vi "Tx to UDP.vi"(6 "Header Details.CustomHeaderLogic":T1, 7 "Data Conversion":T2, 8 "error in (no error)":errorcluster, 10 "Tx Array":dbl[](array[numeric]), 11 "Header Info":bool[](array[boolean])) -> (0 "error out":errorcluster, 1 "payload":dbl[](array[numeric]), 2 "Tx String":string, 5 "Data Conversion out":T2)   [LabVIEW 2019, in "UDP-Custom-Device Engine.lvlib"]
uses:
  UDP-Custom-Device Engine.lvlib
  Types/Engine - Data Conversion Config.ctl
  <vilib>/NI VeriStand/VeriStand Data/Byte Buffer/Byte Buffer.lvclass
  <vilib>/NI VeriStand/VeriStand Data/Byte Buffer/Byte Buffer.Mapping.ctl
  <vilib>/NI VeriStand/VeriStand Data/Typedefs/Typedefs.Data Types.ctl
  Shared/Types/Shared - Custom Header.ctl
  <vilib>/NI VeriStand/VeriStand Data/Byte Buffer/Byte Buffer.lvclass/Byte Buffer.ctl
  <vilib>/NI VeriStand/VeriStand Data/Pointer Operations/Pointer.Write (DBL).vi
  <vilib>/NI VeriStand/VeriStand Data/Byte Buffer/Byte Buffer.Read (String).vi
  <vilib>/NI VeriStand/VeriStand Data/Memory Management/Memory Management.MoveDblBlock.Write (Double).vi
  <vilib>/NI VeriStand/VeriStand Data/Byte Buffer/Byte Buffer.Write.Typed Double Array.vi
  <vilib>/NI VeriStand/VeriStand Data/Utilities/Utilities.Buffer.Double.vi
  <vilib>/NI VeriStand/VeriStand Data/Byte Buffer/Byte Buffer.Subset.Get.vi
  <vilib>/NI VeriStand/VeriStand Data/Byte Buffer/Byte Buffer.Write.vi
  <vilib>/NI VeriStand/VeriStand Data/Byte Buffer/Byte Buffer.Write (1D Boolean).vi
  <vilib>/NI VeriStand/VeriStand Data/Type Conversion/Type Conversion.From Double.Subset.vi
  <vilib>/NI VeriStand/VeriStand Data/Type Conversion/Type Conversion.From Double.Subset (1D Boolean).vi
  <vilib>/NI VeriStand/VeriStand Data/Byte Buffer/Byte Buffer.Write (1D SGL).vi
  <vilib>/NI VeriStand/VeriStand Data/Type Conversion/Type Conversion.From Double.Subset (1D SGL).vi
  <vilib>/NI VeriStand/VeriStand Data/Byte Buffer/Byte Buffer.Write (1D DBL).vi
  <vilib>/NI VeriStand/VeriStand Data/Byte Buffer/Byte Buffer.Write (1D I8).vi
  <vilib>/NI VeriStand/VeriStand Data/Type Conversion/Type Conversion.From Double.Subset (1D I8).vi
  <vilib>/NI VeriStand/VeriStand Data/Byte Buffer/Byte Buffer.Write (1D I16).vi
  <vilib>/NI VeriStand/VeriStand Data/Type Conversion/Type Conversion.From Double.Subset (1D I16).vi
  <vilib>/NI VeriStand/VeriStand Data/Byte Buffer/Byte Buffer.Write (1D I32).vi
  <vilib>/NI VeriStand/VeriStand Data/Type Conversion/Type Conversion.From Double.Subset (1D I32).vi
  <vilib>/NI VeriStand/VeriStand Data/Byte Buffer/Byte Buffer.Write (1D I64).vi
  <vilib>/NI VeriStand/VeriStand Data/Type Conversion/Type Conversion.From Double.Subset (1D I64).vi
  <vilib>/NI VeriStand/VeriStand Data/Byte Buffer/Byte Buffer.Write (1D U8).vi
  <vilib>/NI VeriStand/VeriStand Data/Type Conversion/Type Conversion.From Double.Subset (1D U8).vi
  <vilib>/NI VeriStand/VeriStand Data/Byte Buffer/Byte Buffer.Write (1D U16).vi
  <vilib>/NI VeriStand/VeriStand Data/Type Conversion/Type Conversion.From Double.Subset (1D U16).vi
  <vilib>/NI VeriStand/VeriStand Data/Byte Buffer/Byte Buffer.Write (1D U32).vi
  <vilib>/NI VeriStand/VeriStand Data/Type Conversion/Type Conversion.From Double.Subset (1D U32).vi
  <vilib>/NI VeriStand/VeriStand Data/Byte Buffer/Byte Buffer.Write (1D U64).vi
  <vilib>/NI VeriStand/VeriStand Data/Type Conversion/Type Conversion.From Double.Subset (1D U64).vi
  <vilib>/NI VeriStand/VeriStand Data/Memory Management/Memory Management.MoveByteBlock.Write (String).vi
  <vilib>/NI VeriStand/VeriStand Data/Byte Buffer/Byte Buffer.Get Buffer Pointer.vi
  <vilib>/NI VeriStand/VeriStand Data/Byte Buffer/Byte Buffer.Write (String).vi
  <vilib>/NI VeriStand/VeriStand Data/Type Conversion/Type Conversion.From Double.vi
  <vilib>/NI VeriStand/VeriStand Data/Type Conversion/Type Conversion.From Double (1D Boolean).vi
  <vilib>/NI VeriStand/VeriStand Data/Type Conversion/Type Conversion.From Double (1D SGL).vi
  <vilib>/NI VeriStand/VeriStand Data/Type Conversion/Type Conversion.From Double (1D I8).vi
  <vilib>/NI VeriStand/VeriStand Data/Type Conversion/Type Conversion.From Double (1D I16).vi
  <vilib>/NI VeriStand/VeriStand Data/Type Conversion/Type Conversion.From Double (1D I32).vi
  <vilib>/NI VeriStand/VeriStand Data/Type Conversion/Type Conversion.From Double (1D I64).vi
  <vilib>/NI VeriStand/VeriStand Data/Type Conversion/Type Conversion.From Double (1D U8).vi
  <vilib>/NI VeriStand/VeriStand Data/Type Conversion/Type Conversion.From Double (1D U16).vi
  <vilib>/NI VeriStand/VeriStand Data/Type Conversion/Type Conversion.From Double (1D U32).vi
  <vilib>/NI VeriStand/VeriStand Data/Type Conversion/Type Conversion.From Double (1D U64).vi
  <vilib>/NI VeriStand/VeriStand Data/Byte Buffer/Byte Buffer.Subset.Set.vi
  <vilib>/NI VeriStand/VeriStand Data/Memory Management/Memory Management.MoveByteBlock.Read (String).vi
  <vilib>/NI VeriStand/VeriStand Data/Memory Management/Memory Management.Handle Return.vi
  <vilib>/NI VeriStand/VeriStand Data/Byte Buffer/Byte Buffer.Get Byte Order.vi
  <vilib>/NI VeriStand/VeriStand Data/VeriStand Data.lvlib
  Shared/UDP-Custom-Device Shared.lvlib
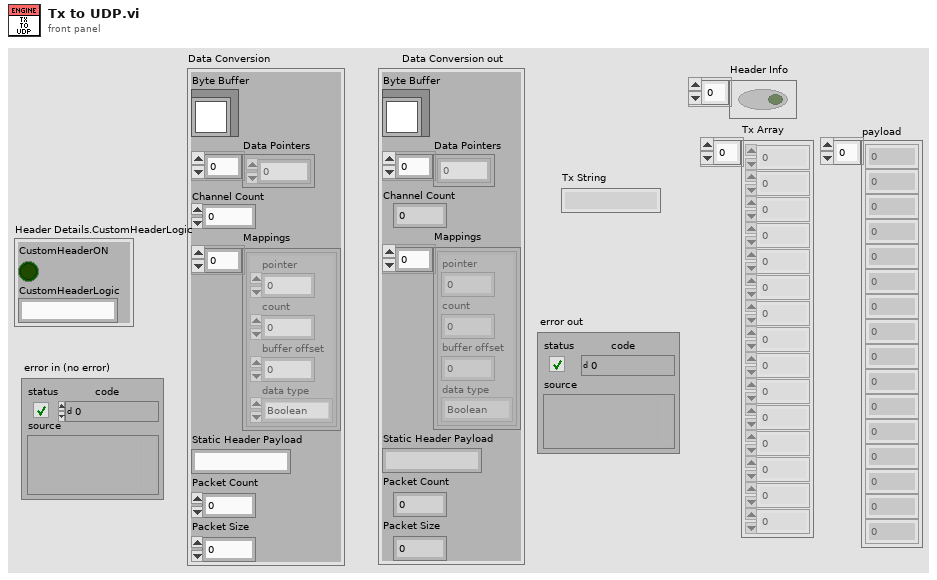
[diagram p1: front panel]
types:
  T1 = typedef "UDP-Custom-Device Shared.lvlib/Shared - Custom Header.ctl" = cluster{"CustomHeaderON":bool, "CustomHeaderLogic":string}
  T2 = typedef "UDP-Custom-Device Engine.lvlib/Engine - Data Conversion Config.ctl" = cluster{"Byte Buffer":refnum<class "Byte Buffer.lvclass">, "Data Pointers":u64[], "Channel Count":i32, "Mappings":T3[], "Static Header Payload":string, "Packet Count":dbl, "Packet Size":i32}
  T3 = typedef "VeriStand Data.lvlib/Byte Buffer.lvclass/Byte Buffer.Mapping.ctl" = cluster{"pointer":u64, "count":i64, "buffer offset":u64, "data type":T4}
  T4 = typedef "VeriStand Data.lvlib/Typedefs.Data Types.ctl" = enum16{"Boolean", "Single", "Double", "I8", "I16", "I32", "I64", "U8", "U16", "U32", "U64"}
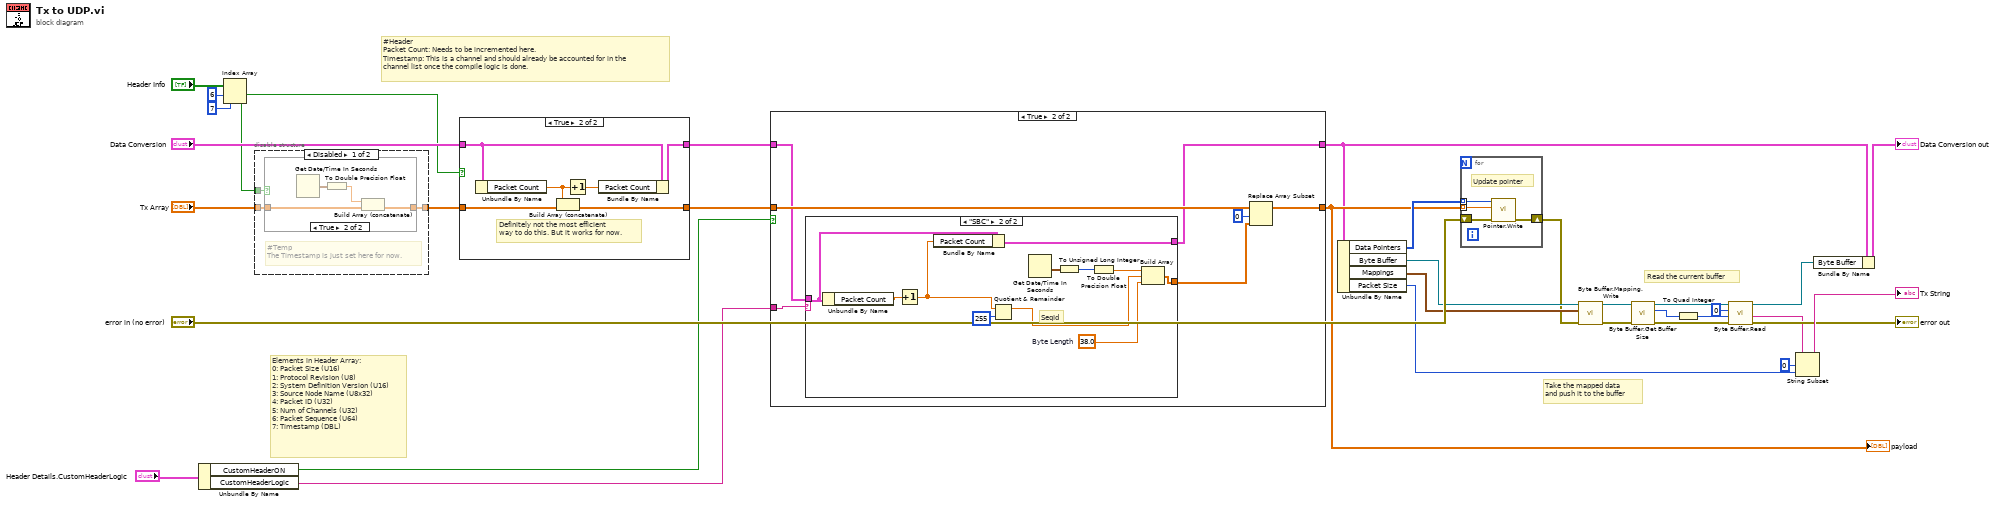
[diagram p0: block diagram]
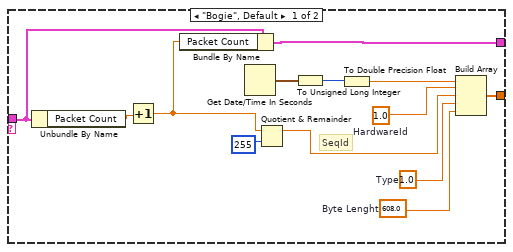
[diagram p3: hidden frame]
diagram:
  # "Elements in Header Array:\n0: Packet Size (U16)\n1: Protocol Revision (U8)\n2: System Definition Version (U16)\n3: Source Node Name (U8x32)\n4: Packet ID (U32)\n5: Num of Channels (U32)\n6: Packet Sequence (U64)\n7: Timestamp (DBL)"
  # "Read the current buffer"
  # "Take the mapped data\nand push it to the buffer"
  # "#Header\nPacket Count: Needs to be incremented here.\nTimestamp: This is a channel and should already be accounted for in the\nchannel list once the compile logic is done."
  n1 = Unbundle By Name("Header Details.CustomHeaderLogic") -> ("CustomHeaderON"=w6:bool, "CustomHeaderLogic"=w5:string)
  n2 = Index Array(array="Header Info", index #1=6 ("index"), index #2=7 ("index")) -> (element #1=w25:bool, element #2=w24:bool)
  n3 = disable-structure shown="Disabled" {
    disable-tunnel: w24 -> [w37 _]
    disable-tunnel: "Tx Array" -> [w36 w43]
    disable-tunnel: [w35 w43] -> w22
    frame Disabled {
      # "#Temp\nThe Timestamp is just set here for now."
      n4 = case shown="True" w37 {
        tunnel: [w38 w41] -> w35
        tunnel: w36 -> [w38 w42]
        frame False {
        }
        frame True {
          n5 = Get Date/Time In Seconds() -> (seconds since 1Jan1904=w40:timestamp)
          n6 = To Double Precision Float(number=w40) -> (double precision float=w39:dbl)
          n7 = Build Array (concatenate)(w39, w42) -> (w41:dbl[])
        }
      }
    }
    frame Enabled {
      # "Timestamp is an input channel\nat compile."
    }
  }
  n8 = case shown="True" w25 {
    tunnel: "Data Conversion" -> [w45 w51]
    tunnel: [w45 w50] -> w2
    tunnel: [w44 w46] -> w4
    tunnel: w22 -> [w44 w47]
    frame False {
    }
    frame True {
      # "Definitely not the most efficient\nway to do this. But it works for now."
      n9 = Unbundle By Name(w51) -> ("Packet Count"=w48:dbl)
      n10 = Build Array (concatenate)(w48, w47) -> (w46:dbl[])
      n11 = Increment(x=w48) -> (x+1=w49:dbl)
      n12 = Bundle By Name(cluster=w51, "Packet Count"=w49) -> (w50:T2)
    }
  }
  n13 = case shown="True" w6 {
    tunnel: w5 -> [_ w59]
    tunnel: w4 -> [w53 w57]
    tunnel: [w53 w60] -> w3
    tunnel: w2 -> [w52 w55]
    tunnel: [w52 w54] -> w1
    frame False {
    }
    frame True {
      n14 = case shown="\"SBC\"" w59 {
        tunnel: [w73 w84] -> w58
        tunnel: w55 -> [w69 w80]
        tunnel: [w68 w79] -> w54
        frame "Bogie", Default {
          w65 = 608.0  # Byte Lenght
          w66 = 1.0  # Type
          w67 = 1.0  # HardwareId
          # "SeqId"
          n15 = Unbundle By Name(w69) -> ("Packet Count"=w70:dbl)
          n16 = Increment(x=w70) -> (x+1=w64:dbl)
          n17 = Bundle By Name(cluster=w69, "Packet Count"=w64) -> (w68:T2)
          n18 = Get Date/Time In Seconds() -> (seconds since 1Jan1904=w63:timestamp)
          n19 = Quotient & Remainder(x=w64, y=u8 255) -> (x-y*floor(x/y)=w71:dbl)  [unwired: 1 out]
          n20 = To Unsigned Long Integer(number=w63) -> (unsigned 32bit integer=w62:u32)
          n21 = To Double Precision Float(number=w62) -> (double precision float=w61:dbl)
          n22 = Build Array(w61, w67, w71, w66, w65) -> (w73:dbl[])
        }
        frame "SBC" {
          w78 = 38.0  # Byte Length
          # "SeqId"
          n23 = Unbundle By Name(w80) -> ("Packet Count"=w81:dbl)
          n24 = Increment(x=w81) -> (x+1=w77:dbl)
          n25 = Bundle By Name(cluster=w80, "Packet Count"=w77) -> (w79:T2)
          n26 = Quotient & Remainder(x=w77, y=u8 255) -> (x-y*floor(x/y)=w82:dbl)  [unwired: 1 out]
          n27 = Get Date/Time In Seconds() -> (seconds since 1Jan1904=w75:timestamp)
          n28 = To Unsigned Long Integer(number=w75) -> (unsigned 32bit integer=w76:u32)
          n29 = To Double Precision Float(number=w76) -> (double precision float=w74:dbl)
          n30 = Build Array(w74, w82, w78) -> (w84:dbl[])
        }
      }
      n31 = Replace Array Subset(array=w57, new element=w58, index=0) -> (w60:dbl[])
    }
  }
  "payload" <- w3
  n32 = Unbundle By Name(w1) -> ("Data Pointers"=w32:u64[], "Byte Buffer"=w30:refnum<class "Byte Buffer.lvclass">, "Mappings"=w31:T3[], "Packet Size"=w19:i32)
  n33 = for {
    tunnel: w32 -> [w87] mode=indexing
    tunnel: w3 -> [w85] mode=indexing
    shift-right: [w86] -> w29
    shift-left: "error in (no error)" -> [w88]
    # "Update pointer"
    n34 = call-poly <vilib>:"Pointer.Write.vi"("error in (no error)"=w88, "value"=w85, "pointer in"=w87) -> ("error out"=w86:errorcluster)  [unwired: 6 in, 2 out]
  }
  n35 = call <vilib>:"Byte Buffer.Mapping.Write.vi"("error in (no error)"=w29, "mappings"=w31, "Byte Buffer in"=w30) -> ("error out"=w12:errorcluster, "Byte Buffer out"=w14:refnum<class "Byte Buffer.lvclass">)  [unwired: 6 in, 1 out]
  n36 = call <vilib>:"Byte Buffer.Get Buffer Size.vi"("error in (no error)"=w12, "Byte Buffer in"=w14) -> ("error out"=w11:errorcluster, "buffer size"=w10:u64, "Byte Buffer out"=w13:refnum<class "Byte Buffer.lvclass">)  [unwired: 7 in]
  n37 = To Quad Integer(1:w10) -> (0:w9:i64)
  n38 = call-poly <vilib>:"Byte Buffer.Read.vi"("error in (no error)"=w11, "size"=w9, "buffer offset"=u64 0, "Byte Buffer in"=w13) -> ("error out"=→"error out":errorcluster, "string"=w15:string, "Byte Buffer out"=w17:refnum<class "Byte Buffer.lvclass">)  [unwired: 4 in, 1 out]
  n39 = String Subset(string=w15, offset (0)=0, length (rest)=w19) -> (substring=→"Tx String":string)
  n40 = Bundle By Name(cluster=w1, "Byte Buffer"=w17) -> (→"Data Conversion out":T2)
